vi "InsertBlockData.vi"(0 "C12LE":dbl, 1 "C12":dbl, 2 "Block Data In":T1, 5 "C13H":dbl, 7 "C13L":dbl, 9 "C13LE":dbl, 11 "Counts":u32, 12 "LT":dbl, 13 "RT":dbl) -> (4 "Block Data Out":T1)   [LabVIEW 2013]
uses:
  ctl/BlockData.ctl
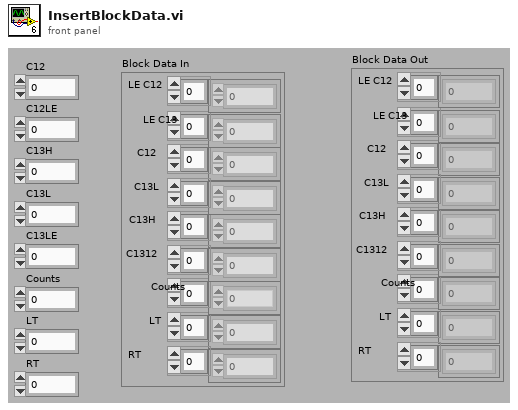
[diagram p1: front panel]
types:
  T1 = typedef "BlockData.ctl" = cluster{"LE C12":dbl[], "LE C13":dbl[], "C12":dbl[], "C13L":dbl[], "C13H":dbl[], "C1312":dbl[], "Counts":u32[], "LT":dbl[], "RT":dbl[]}
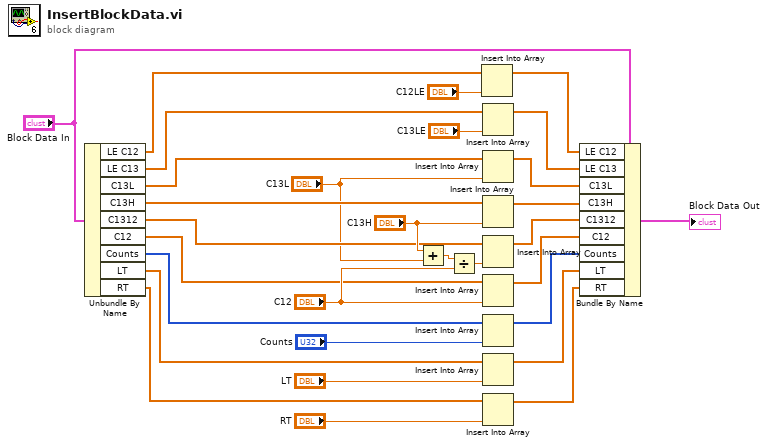
[diagram p0: block diagram]
diagram:
  n1 = Unbundle By Name("Block Data In") -> ("LE C12"=w6:dbl[], "LE C13"=w4:dbl[], "C13L"=w13:dbl[], "C13H"=w10:dbl[], "C1312"=w12:dbl[], "C12"=w11:dbl[], "Counts"=w28:u32[], "LT"=w27:dbl[], "RT"=w26:dbl[])
  n2 = Add(x="C13H", y="C13L") -> (x+y=w19:dbl)
  n3 = Divide(x=w19, y="C12") -> (x/y=w18:dbl)
  n4 = Insert Into Array(array=w6, new element="C12LE") -> (w5:dbl[])  [unwired: 1 in]
  n5 = Insert Into Array(array=w4, new element="C13LE") -> (w3:dbl[])  [unwired: 1 in]
  n6 = Insert Into Array(array=w13, new element="C13L") -> (w14:dbl[])  [unwired: 1 in]
  n7 = Insert Into Array(array=w10, new element="C13H") -> (w15:dbl[])  [unwired: 1 in]
  n8 = Insert Into Array(array=w12, new element=w18) -> (w16:dbl[])  [unwired: 1 in]
  n9 = Insert Into Array(array=w11, new element="C12") -> (w17:dbl[])  [unwired: 1 in]
  n10 = Insert Into Array(array=w28, new element="Counts") -> (w25:u32[])  [unwired: 1 in]
  n11 = Insert Into Array(array=w27, new element="LT") -> (w24:dbl[])  [unwired: 1 in]
  n12 = Insert Into Array(array=w26, new element="RT") -> (w23:dbl[])  [unwired: 1 in]
  n13 = Bundle By Name(cluster="Block Data In", "LE C12"=w5, "LE C13"=w3, "C13L"=w14, "C13H"=w15, "C1312"=w16, "C12"=w17, "Counts"=w25, "LT"=w24, "RT"=w23) -> (→"Block Data Out":T1)
